vi "Configure Initiate Continous [CA] Core.vi"(8 "error in (no error)":errorcluster, 10 "continuous acquisition (Disabled)":bool, 11 "CS++Scope":refnum<class "CS++Scope.lvclass">) -> (0 "error out":errorcluster, 3 "CS++Scope out":refnum<class "CS++Scope.lvclass">)   [LabVIEW 2016, in "CS++Scope.lvlib" / "CS++Scope.lvclass"]
doc: "This VI configures the oscilloscope to perform continuous acquisition."
uses:
  CS++Scope.lvclass
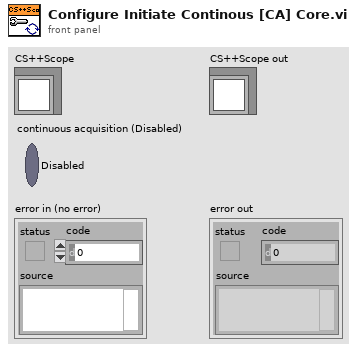
[diagram p1: front panel]
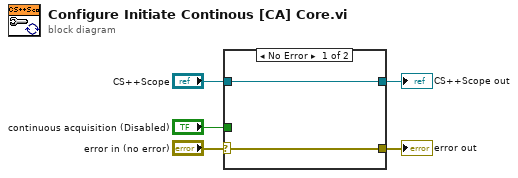
[diagram p0: block diagram]
diagram:
  n1 = case shown="No Error" "error in (no error)" {
    selector: "error in (no error)" -> [w6 w9]
    tunnel: [w6 w9] -> w4
    tunnel: [w7 w8] -> w1
    tunnel: "CS++Scope" -> [w7 w8]
    tunnel: "continuous acquisition (Disabled)" -> [_ _]
    frame No Error {
    }
    frame Error {
    }
  }
  "error out" <- w4
  "CS++Scope out" <- w1
